vi "SPD.Set Temp and Wait For Ready.vi"(7 "Continue":refnum<vi>, 8 "Error In":errorcluster, 10 "Tset":dbl, 11 "SPD.Stand Ctrl in":T1 {"spdDeviceSession"."hidSPD.Sturtup Values"."HV_bias" format="%#_6p, V"; "spdDeviceSession"."hidSPD.Sturtup Values"."TSet" format="%#_6p, DegC"; "spdDeviceSession"."hidSPD.Controller"."HV_bias" format="%#_6p, V"; "spdDeviceSession"."hidSPD.Controller"."TSet" format="%#_6p, DegC"}) -> (0 "Error Out":errorcluster, 3 "SPD.Stand Ctrl out":T1 {"spdDeviceSession"."hidSPD.Sturtup Values"."HV_bias" format="%#_6p, V"; "spdDeviceSession"."hidSPD.Sturtup Values"."TSet" format="%#_6p, DegC"; "spdDeviceSession"."hidSPD.Controller"."HV_bias" format="%#_6p, V"; "spdDeviceSession"."hidSPD.Controller"."TSet" format="%#_6p, DegC"})   [LabVIEW 2018]
uses:
  typedefs/SPD.Stand Ctrl.ctl
  Instruments/SPD HID Interface/hidSPDLibForLabView/LibVIs/hidSPD Controls/hidSPD Device Session.ctl
  Instruments/SPD HID Interface/hidSPDLibForLabView/LibVIs/hidSPD Controls/hidSPD Controller.ctl
  Instruments/SPD HID Interface/hidSPDLibForLabView/LibVIs/hidSPD Controls/hidSPD SPD Type.ctl
  Instruments/KC705 DevBoard/typedefs/DevB.Session.ctl
  Instruments/KeySight 53230A/typedefs/FreqC.Session.ctl
  Instruments/KeySight 8164B/KeySight 8164B LAN InstrLib/typedefs/KeySight 8164B control.ctl
  Instruments/LeCroy SDA830/typedefs/LeCroy.Session.ctl
  typedefs/SPD.Events.ctl
  ConfigFile/SPD.Config File ctrl.ctl
  <vilib>/Utility/config.llb/Config Data RefNum.ctl
  typedefs/SPD.Meas Result.ctl
  typedefs/SPD.Queues.ctl
  typedefs/SPD.Stand state.ctl
  Instruments/SPD HID Interface/hidSPDLibForLabView/LibVIs/hidSPD Controls/hidSPD Controller Setup Report.ctl
  Instruments/SPD HID Interface/hidSPDLibForLabView/LibVIs/hidSPD Write Report/hidSPD Setup Controller.vi
  Instruments/SPD HID Interface/hidSPDLibForLabView/hidSPDLibForLabView.lvlib
  Instruments/KeySight 8164B/KeySight 8164B LAN InstrLib.lvlib
  <vilib>/Utility/config.llb/NI_LVConfig.lvlib
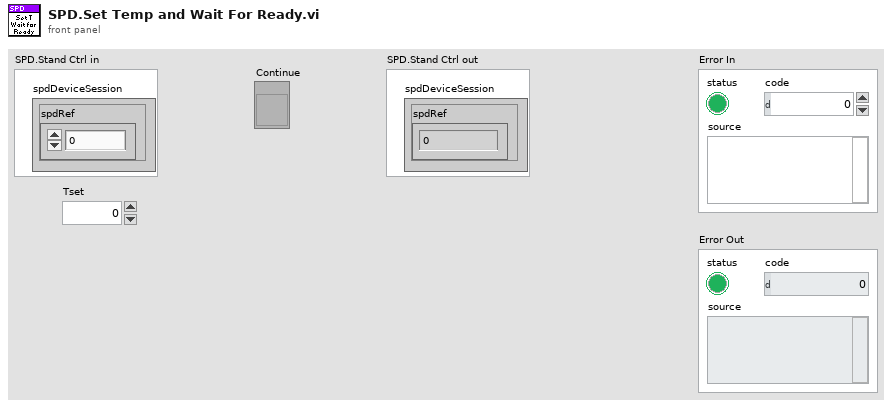
[diagram p1: front panel]
types:
  T1 = typedef "SPD.Stand Ctrl.ctl" = cluster{"spdDeviceSession":T2, "DevBSession":T5, "FreqCSession":T6, "8164BSession":T7, "LeCroySession":T8, "Events":T9, "configFile":T10, "SPD.Result":T12, "SPD.Queues":T13, "Console":refnum<vi>}
  T2 = typedef "hidSPDLibForLabView.lvlib/hidSPD Device Session.ctl" = cluster{"spdRef":u64, "connected":bool, "spdName":string, "hidSPD.Controller":T3, "hidSPD.Sturtup Values":T3, "SPD Type":T4}
  T3 = typedef "hidSPDLibForLabView.lvlib/hidSPD Controller.ctl" = cluster{"TSet":sgl, "HV_bias":sgl, "DDS_stb_code":u16}
  T4 = typedef "hidSPDLibForLabView.lvlib/hidSPD SPD Type.ctl" = enum16{"Free Run", "Strobe"}
  T5 = typedef "DevB.Session.ctl" = cluster{"DevBRef":refnum<visa-resource-name>, "connected":bool}
  T6 = typedef "FreqC.Session.ctl" = cluster{"FreqCRef":refnum<visa-resource-name>, "timeout":dbl, "Gate":dbl, "connected":bool}
  T7 = typedef "KeySight 8164B LAN InstrLib.lvlib/KeySight 8164B control.ctl" = cluster{"Connection ID":refnum<k5>, "Connected":bool, "Info":string, "Slots Info":string[]}
  T8 = typedef "LeCroy.Session.ctl" = cluster{"LeCroySession":refnum<visa-resource-name>, "connected":bool}
  T9 = typedef "SPD.Events.ctl" = cluster{"DCRTest":refnum<user-event>, "Stop":refnum<user-event>}
  T10 = typedef "SPD.Config File ctrl.ctl" = cluster{"configFile ref":T11, "configFile path":path, "equipmentFile ref":T11}
  T11 = typedef "NI_LVConfig.lvlib/Config Data RefNum.ctl" = refnum<k1>
  T12 = typedef "SPD.Meas Result.ctl" = cluster{"HV_Bias":dbl[][][], "Stb_code":dbl[], "Temprature":dbl[], "Data":dbl[][][][], "DateTime":string}
  T13 = typedef "SPD.Queues.ctl" = cluster{"state queue":refnum<queue>}
  T14 = typedef "hidSPDLibForLabView.lvlib/hidSPD Controller Setup Report.ctl" = cluster{"TSet":sgl, "HV_bias":sgl, "DDS_stb_code":u16, "SPD_reset":u16, "MCU_reset":u16}
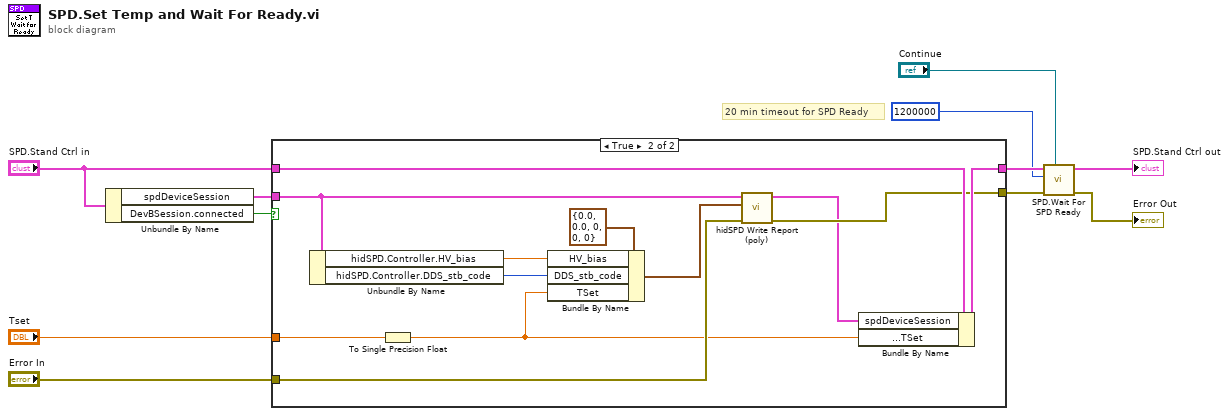
[diagram p0: block diagram]
diagram:
  # "20 min timeout for SPD Ready"
  n1 = Unbundle By Name("SPD.Stand Ctrl in") -> ("spdDeviceSession"=w11:T2, "DevBSession.connected"=w10:bool)
  n2 = case shown="True" w10 {
    tunnel: w11 -> [_ w21]
    tunnel: "Error In" -> [w12 w23]
    tunnel: "SPD.Stand Ctrl in" -> [w13 w25]
    tunnel: [w13 w24] -> w2
    tunnel: [w12 w22] -> w6
    tunnel: "Tset" -> [_ w16]
    frame False {
    }
    frame True {
      n3 = Unbundle By Name(w21) -> ("hidSPD.Controller.HV_bias"=w18:sgl, "hidSPD.Controller.DDS_stb_code"=w17:u16)
      n4 = To Single Precision Float(number=w16) -> (single precision float=w15:sgl)
      n5 = Bundle By Name(cluster=T14 {"TSet"=0.0, "HV_bias"=0.0, "DDS_stb_code"=0, "SPD_reset"=0, "MCU_reset"=0} ("hidSPD Controller Setup report"), "HV_bias"=w18, "DDS_stb_code"=w17, "TSet"=w15) -> (w19:T14)
      n6 = call-poly "hidSPD Write Report (poly).vi"("error in (no error)"=w23, "hidSPD Controller Setup report"=w19, "spdDevSession in"=w21) -> ("error out"=w22:errorcluster, "spdDevSession out"=w14:T2)  [unwired: 7 in]
      n7 = Bundle By Name(cluster=w25, "spdDeviceSession"=w14, "spdDeviceSession.hidSPD.Controller.TSet"=w15) -> (w24:T1)
    }
  }
  n8 = call "SPD.Wait For SPD Ready.vi"("Continue"="Continue", "Error In"=w6, "timeout (ms)"=u32 1200000, "SPD.Stand Ctrl in"=w2) -> ("Error Out"=→"Error Out":errorcluster, "SPD.Stand Ctrl out"=→"SPD.Stand Ctrl out":T1)  [unwired: 6 in]
